vi "Disconnect.vi"(8 "Error In":errorcluster, 10 "Resource Name":refnum<k15>, 11 "object in":refnum<class "Disconnected.lvclass">) -> (0 "Error Out":errorcluster, 3 "object out":refnum<class "IStates.lvclass">)   [LabVIEW 2023, in "PXI-5441.lvlib" / "Disconnected.lvclass"]
uses:
  Disconnected.lvclass
  IScope_interface/IStates_interface/IStates.lvclass
  Disconnected.lvclass/Disconnected.ctl
  D:/git/HAL/PXI-5441_class/states/Disconnected_class/Disconnected.lvclass
  D:/git/HAL/IScope_interface/IStates_interface/IStates.lvclass
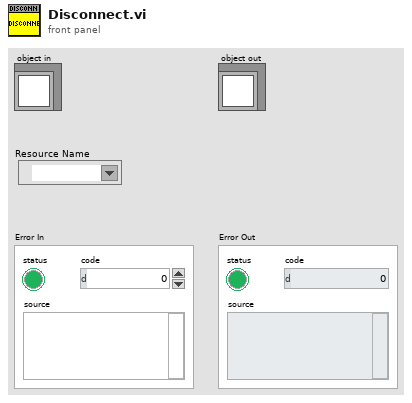
[diagram p1: front panel]
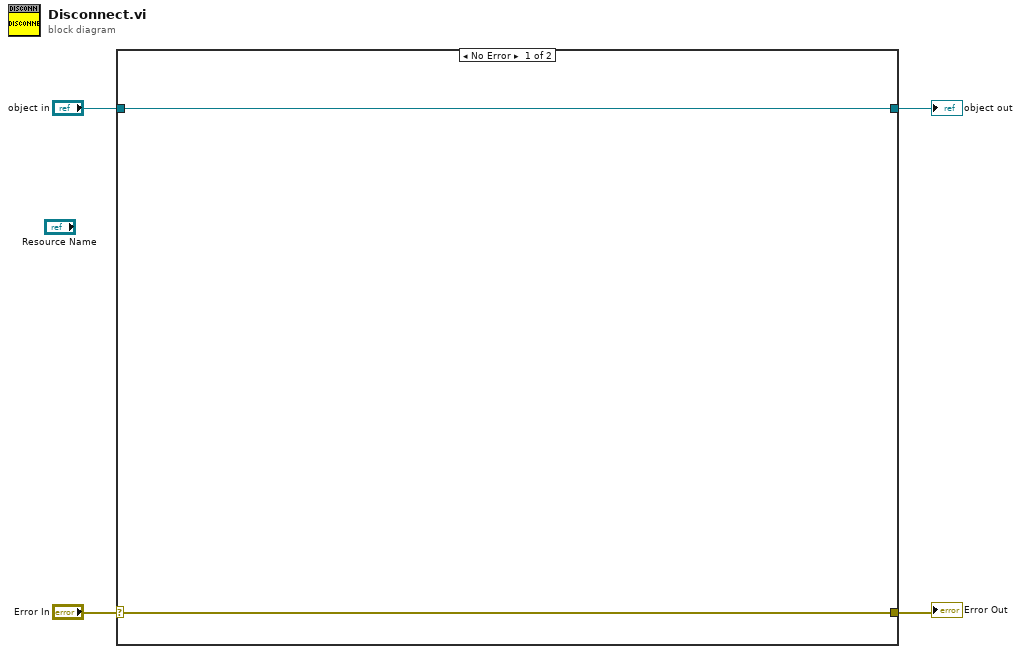
[diagram p0: block diagram]
diagram:
  n1 = case shown="No Error" "Error In" {
    selector: "Error In" -> [w6 w8]
    tunnel: [w6 w8] -> w3
    tunnel: [w5 w7] -> w1
    tunnel: "object in" -> [w5 w7]
    frame No Error {
    }
    frame Error {
    }
  }
  "Error Out" <- w3
  "object out" <- w1
